vi "Calc time of measurement NPLs.vi"(1 "Number of Power Line Cycles(50Hz)":dbl=50.0, 2 "2182 -A Params":T1={"Auto Range?"=FALSE, "Man / Selected\n       Range"=enum."10mV", "Enable Digital\n       Filter?"=FALSE, "Filter Type"=enum."Movin", "Filter Count"=1, "      Filter\nWindow (%)"=0.01, "Enable Analog\n       Filter?"=FALSE, "NPLCs"=5} {"NPLCs" min=1 max=10; "Filter\nWindow (%)" min=0.01 max=10.0 step=0.01 format="%.2f"; "Filter Count" min=1 max=100}) -> (0 "Time of one measurement":dbl=7100.0)   [LabVIEW 2013, in "Keithly user program.lvlib"]
uses:
  Keithly user program.lvlib
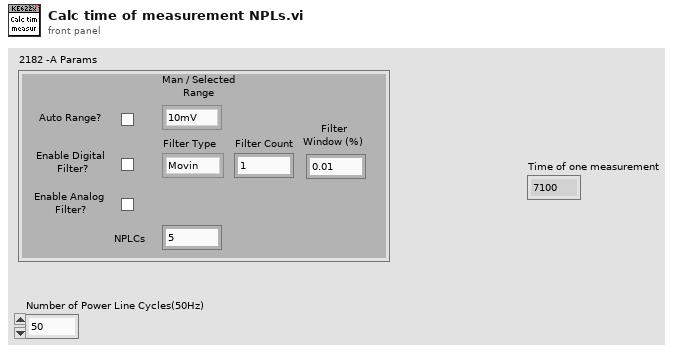
[diagram p1: front panel]
types:
  T1 = cluster{"Auto Range?":bool, "Man / Selected\n       Range":enum16{"10mV", "100mV", "1V", "10V", "100V"}, "Enable Digital\n       Filter?":bool, "Filter Type":enum16{"Movin", "Repeat"}, "Filter Count":u32, "      Filter\nWindow (%)":dbl, "Enable Analog\n       Filter?":bool, "NPLCs":u32}
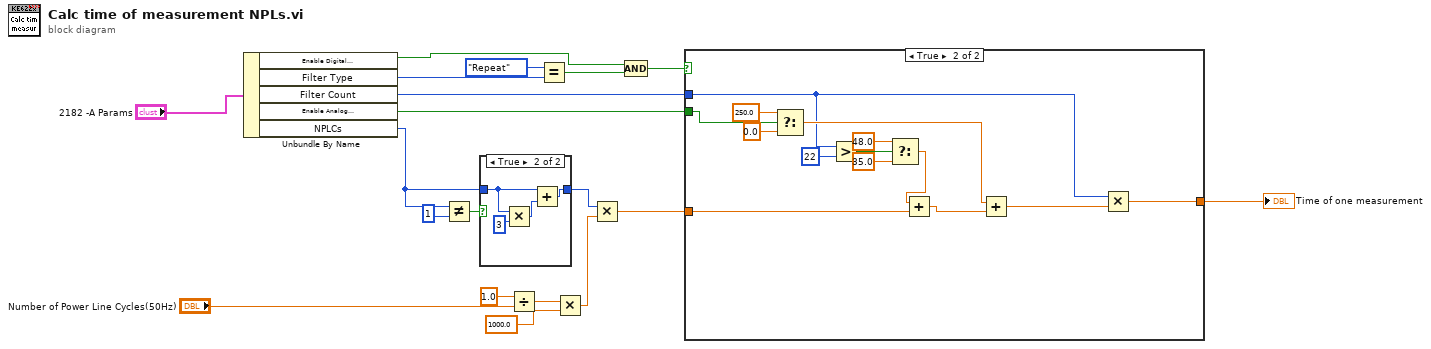
[diagram p0: block diagram]
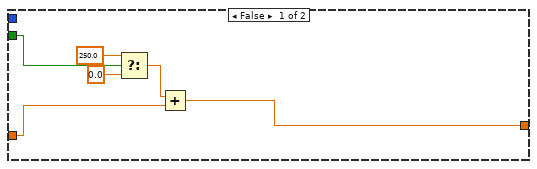
[diagram p2: hidden frame]
diagram:
  n1 = Unbundle By Name("2182 -A Params") -> ("Enable Digital\n       Filter?"=w8:bool, "Filter Type"=w10:enum16{"Movin", "Repeat"}, "Filter Count"=w4:u32, "Enable Analog\n       Filter?"=w1:bool, "NPLCs"=w2:u32)
  n2 = Not Equal?(x=w2, y=u32 1) -> (x != y?=w18:bool)
  n3 = case shown="True" w18 {
    tunnel: w2 -> [w20 w22]
    tunnel: [w20 w24] -> w19
    frame False {
    }
    frame True {
      n4 = Multiply(x=w22, y=u32 3) -> (x*y=w23:u32)
      n5 = Add(x=w22, y=w23) -> (x+y=w24:u32)
    }
  }
  n6 = Divide(x=1.0, y="Number of Power Line Cycles(50Hz)") -> (x/y=w14:dbl)
  n7 = Equal?(x=enum16{"Movin", "Repeat"}."Repeat", y=w10) -> (x = y?=w7:bool)
  n8 = Multiply(x=w14, y=1000.0) -> (x*y=w16:dbl)
  n9 = Multiply(x=w19, y=w16) -> (x*y=w5:dbl)
  n10 = Compound Arithmetic op=AND(w8, w7) -> (w6:bool)
  n11 = case shown="True" w6 {
    tunnel: w5 -> [w27 w38]
    tunnel: w4 -> [_ w36]
    tunnel: [w25 w44] -> w3
    tunnel: w1 -> [w28 w43]
    frame False {
      n12 = Select(t=250.0, s=w28, f=0.0) -> (s? t:f=w26:dbl)
      n13 = Add(x=w26, y=w27) -> (x+y=w25:dbl)
    }
    frame True {
      n14 = Select(t=250.0, s=w43, f=0.0) -> (s? t:f=w40:dbl)
      n15 = Greater?(x=w36, y=u32 22) -> (0:w34:bool)
      n16 = Select(t=48.0, s=w34, f=35.0) -> (s? t:f=w31:dbl)
      n17 = Add(x=w31, y=w38) -> (x+y=w37:dbl)
      n18 = Add(x=w40, y=w37) -> (x+y=w39:dbl)
      n19 = Multiply(x=w36, y=w39) -> (x*y=w44:dbl)
    }
  }
  "Time of one measurement" <- w3
